vi "DetermineSpeedCap.vi"(2 "Speed Cap Decceleration Limit (ft/s^2)":dbl=15.0, 3 "Driver Profile Doesn't Want to Shift":bool, 4 "Master State In":T1(ring)) -> (0 "Speed Cap [0,1]":dbl)   [LabVIEW 2023]
doc: "Determines the speed cap for the swerve drive based on the control inputs and master alarms. This includes forcing the robot into low gear."
uses:
  GlobalDriverStationCommands.vi
  GlobalDrivebase.vi
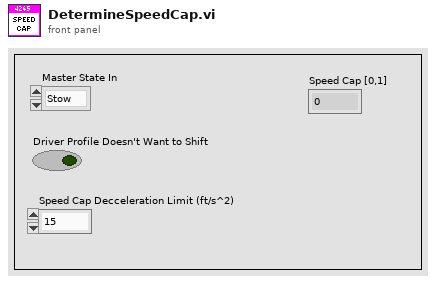
[diagram p1: front panel]
types:
  T1 = enum16{"Stow", "Speaker", "Amp", "Climbing", "Trap"}
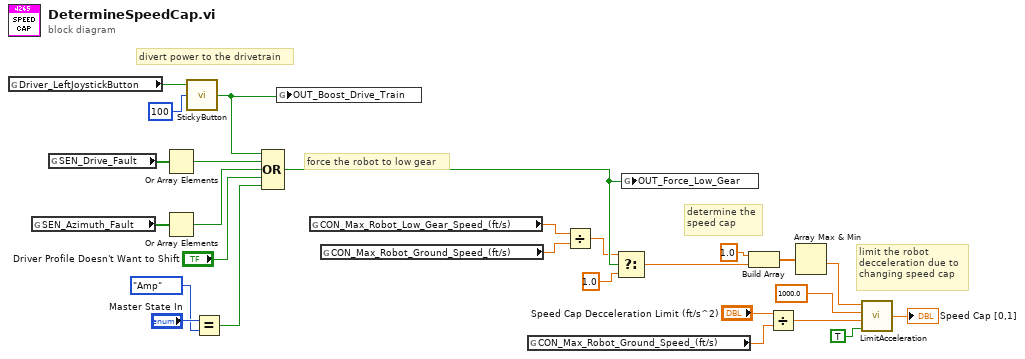
[diagram p0: block diagram]
diagram:
  # "limit the robot\ndecceleration due to\nchanging speed cap"
  # "force the robot to low gear"
  # "determine the\nspeed cap"
  # "divert power to the drivetrain"
  n1 = global read "GlobalDriverStationCommands.vi" "Driver_LeftJoystickButton"() -> (w10:bool)
  n2 = global read "GlobalDrivebase.vi" "SEN_Azimuth_Fault"() -> (w26:bool[])
  n3 = global read "GlobalDrivebase.vi" "SEN_Drive_Fault"() -> (w6:bool[])
  n4 = Or Array Elements(Boolean array=w6) -> (logical OR=w5:bool)
  n5 = Or Array Elements(Boolean array=w26) -> (logical OR=w13:bool)
  n6 = call "StickyButton.vi"("Time threshold (ms)"=u32 100 ("y"), "Button Input"=w10) -> ("Sticky Button"=w4:bool)  [unwired: 1 in]
  n7 = Equal?(x="Master State In", y=T1."Amp") -> (x = y?=w1:bool)
  n8 = Compound Arithmetic op=OR(w4, w5, w13, "Driver Profile Doesn't Want to Shift", w1) -> (w25:bool)
  n9 = global write "GlobalDrivebase.vi" "OUT_Boost_Drive_Train"(w4) -> ()
  n10 = global read "GlobalDrivebase.vi" "CON_Max_Robot_Low_Gear_Speed_(ft/s)"() -> (w23:dbl)
  n11 = global read "GlobalDrivebase.vi" "CON_Max_Robot_Ground_Speed_(ft/s)"() -> (w24:dbl)
  n12 = global read "GlobalDrivebase.vi" "CON_Max_Robot_Ground_Speed_(ft/s)"() -> (w8:dbl)
  n13 = Divide(x=w23, y=w24) -> (x/y=w20:dbl)
  n14 = Select(t=w20, s=w25, f=1.0) -> (s? t:f=w21:dbl)
  n15 = global write "GlobalDrivebase.vi" "OUT_Force_Low_Gear"(w25) -> ()
  n16 = Build Array(1.0 ("element"), w21) -> (w14:dbl[])
  n17 = Divide(x="Speed Cap Decceleration Limit (ft/s^2)", y=w8) -> (x/y=w7:dbl)
  n18 = Array Max & Min(array=w14) -> (min value=w17:dbl)  [unwired: 3 out]
  n19 = call "LimitAcceleration.vi"("Apply Limit"=TRUE, "Decceleration Limit (/s)"=w7, "Acceleration Limit (/s)"=1000.0, "Raw Input"=w17) -> ("Output"=→"Speed Cap [0,1]":dbl)
